vi "Process.vi"(8 "error in (no error)":errorcluster, 10 "Update Wash Display Console Msg in":refnum<class "Update Wash Display Console Msg.lvclass">, 11 "Architecture.lvlib:Thread.lvclass":refnum<class "Thread.lvclass">) -> (0 "error out":errorcluster, 1 "Stop?":bool, 3 "Architecture.lvlib:Thread.lvclass 2":refnum<class "Thread.lvclass">)   [LabVIEW 2016, in "Wash Display Console.lvlib" / "Update Wash Display Console Msg.lvclass"]
uses:
  Update Wash Display Console Msg.lvclass
  Wash Display Console/Wash Display Console.lvclass
  C:/Users/nitest/Downloads/Sample Exams/Carwash (100529-01)/Actor Objects/Thread/Thread.lvclass
  Thread/Thread.lvclass
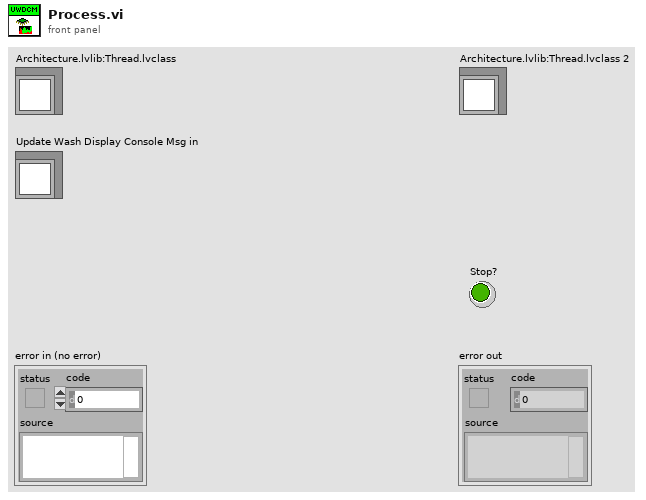
[diagram p1: front panel]
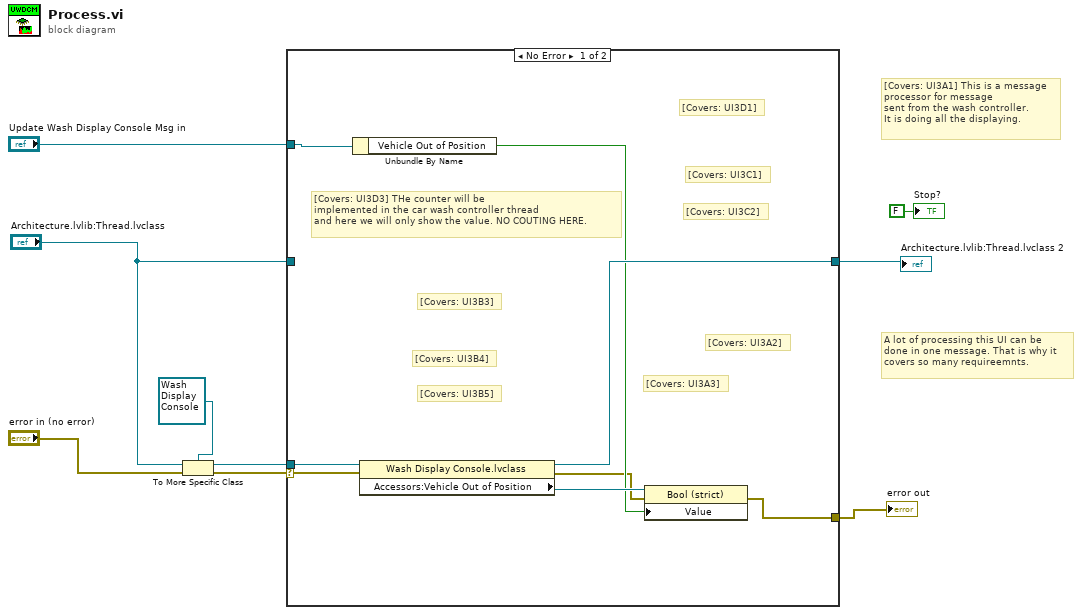
[diagram p0: block diagram]
diagram:
  # "A lot of processing this UI can be\ndone in one message. That is why it\ncovers so many requireemnts."
  # "[Covers: UI3A1] This is a message\nprocessor for message\nsent from the wash controller.\nIt is doing all the displaying."
  n1 = To More Specific Class(target class=refnum<class "Wash Display Console.lvclass"> refnum ("Wash Display Console.lvlib:Wash Display Console.lvclass"), reference="Architecture.lvlib:Thread.lvclass", error in="error in (no error)") -> (specific class reference=w7:refnum<class "Wash Display Console.lvclass">, error out=w8:errorcluster)
  n2 = case shown="No Error" w8 {
    selector: w8 -> [w16 w18]
    tunnel: w7 -> [w17 _]
    tunnel: [w14 w19] -> w4
    tunnel: "Architecture.lvlib:Thread.lvclass" -> [_ w19]
    tunnel: [w11 w18] -> w2
    tunnel: "Update Wash Display Console Msg in" -> [w13 _]
    frame No Error {
      # "[Covers: UI3D3] THe counter will be\nimplemented in the car wash controller thread\nand here we will only show the value. NO COUTING HERE."
      # "[Covers: UI3D1]"
      # "[Covers: UI3C2]"
      # "[Covers: UI3C1]"
      # "[Covers: UI3B5]"
      # "[Covers: UI3B4]"
      # "[Covers: UI3B3]"
      # "[Covers: UI3A3]"
      # "[Covers: UI3A2]"
      n3 = Unbundle By Name(w13) -> ("Vehicle Out of Position"=w12:bool)
      n4 = property class="Wash Display Console.lvclass"(reference=w17, error in=w16) -> (reference out=w14:refnum<class "Wash Display Console.lvclass">, error out=w10:errorcluster, "Accessors:Vehicle Out of Position"=w15:refnum<vi>)
      n5 = property class="Bool (strict)"(reference=w15, error in=w10, "Value"=w12) -> (error out=w11:errorcluster)  [unwired: 1 out]
    }
    frame Error {
    }
  }
  "error out" <- w2
  "Architecture.lvlib:Thread.lvclass 2" <- w4
  "Stop?" <- FALSE ("Stop?")
